vi "Path to LV File Type.vi"(11 "path":path) -> (0 "lvlibp":bool, 1 "llb":bool, 2 "ctl":bool, 3 "vi":bool, 4 "lvproj":bool, 5 "lvlib":bool)   [LabVIEW 2015]
doc: "Returns LV file type based on file extension."
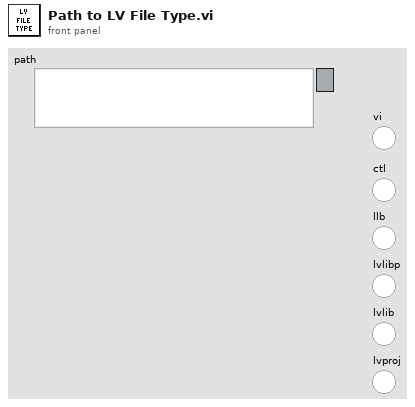
[diagram p1: front panel]
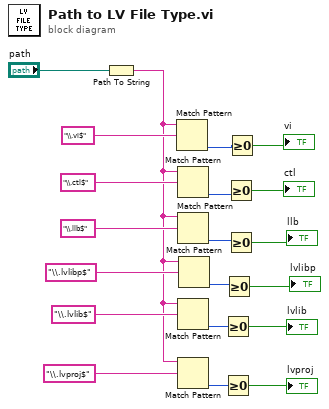
[diagram p0: block diagram]
diagram:
  n1 = Path To String(path="path") -> (string=w1:string)
  n2 = Match Pattern(string=w1, regular expression="\\.vi$") -> (offset past match=w18:i32)  [unwired: 1 in, 3 out]
  n3 = Match Pattern(string=w1, regular expression="\\.ctl$") -> (offset past match=w12:i32)  [unwired: 1 in, 3 out]
  n4 = Match Pattern(string=w1, regular expression="\\.llb$") -> (offset past match=w9:i32)  [unwired: 1 in, 3 out]
  n5 = Match Pattern(string=w1, regular expression="\\.lvlib$") -> (offset past match=w6:i32)  [unwired: 1 in, 3 out]
  n6 = Match Pattern(string=w1, regular expression="\\.lvproj$") -> (offset past match=w3:i32)  [unwired: 1 in, 3 out]
  n7 = Match Pattern(string=w1, regular expression="\\.lvlibp$") -> (offset past match=w8:i32)  [unwired: 1 in, 3 out]
  n8 = Greater Or Equal To 0?(x=w6) -> (x >= 0?=→"lvlib":bool)
  n9 = Greater Or Equal To 0?(x=w3) -> (x >= 0?=→"lvproj":bool)
  n10 = Greater Or Equal To 0?(x=w8) -> (x >= 0?=→"lvlibp":bool)
  n11 = Greater Or Equal To 0?(x=w12) -> (x >= 0?=→"ctl":bool)
  n12 = Greater Or Equal To 0?(x=w9) -> (x >= 0?=→"llb":bool)
  n13 = Greater Or Equal To 0?(x=w18) -> (x >= 0?=→"vi":bool)
